vi "Command Loop - Set HW Values.vi"(8 "error in":errorcluster, 10 "Data":string, 11 "Queue Refs in":variant) -> (0 "error out":errorcluster, 2 "Response":string, 3 "Queue Refs out":variant)   [LabVIEW 2026, in "Runtime Configuration Support Example Engine.lvlib"]
uses:
  Runtime Configuration Support Example Engine.lvlib
  <vilib>/NI VeriStand/Custom Device API/Custom Device Item Ref.ctl
  <vilib>/NI VeriStand/Custom Device API/Custom Device API.lvlib
  Shared/Compiled.Settings.ctl
  Shared/Runtime Configuration Support Example Shared.lvlib
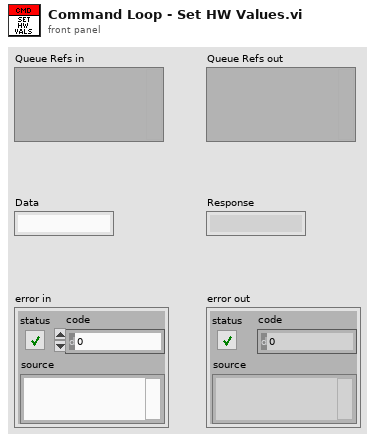
[diagram p1: front panel]
types:
  T1 = cluster{"Compiled Info":refnum<queue>, "Set HW Val Ref":refnum<queue>, "Get HW Val Ref":refnum<queue>}
  T2 = cluster{"SignalIDs":i32[], "Values":i32[], "Response Ref":refnum<queue>}
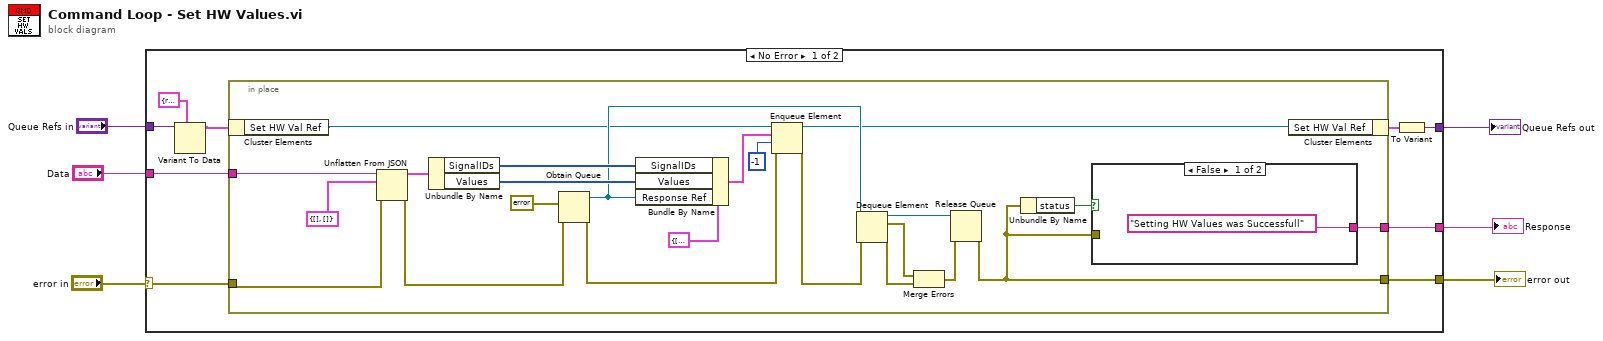
[diagram p0: block diagram]
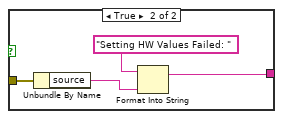
[diagram p2: hidden frame]
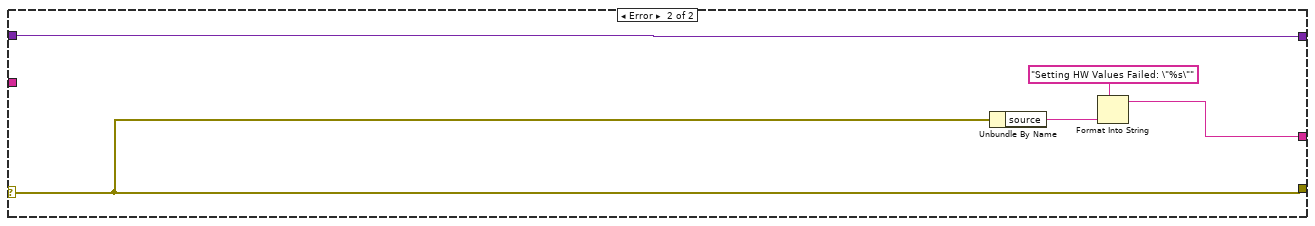
[diagram p3: hidden frame]
diagram:
  n1 = case shown="No Error" "error in" {
    selector: "error in" -> [w15 w48]
    tunnel: "Data" -> [w13 _]
    tunnel: "Queue Refs in" -> [w11 w44]
    tunnel: [w12 w45] -> w3
    tunnel: [w14 w48] -> w5
    tunnel: [w7 w44] -> w1
    frame No Error {
      n2 = Variant To Data(type=T1 {"Compiled Info"=refnum, "Set HW Val Ref"=refnum, "Get HW Val Ref"=refnum} ("Queue Refs in"), Variant=w11) -> (data=w10:T1)  [unwired: 1 in, 1 out]
      n3 = in-place {
        in-place-border: w15 -> [w34]
        in-place-border: [w32] -> w14
        in-place-border: w13 -> [w23]
        in-place-border: [w20] -> w12
        n4 = in-place-cluster #1(w10) -> ("Set HW Val Ref"=w19:refnum<queue>)
        n5 = Unflatten From JSON(JSON string=w23, type and defaults=cluster{"SignalIDs":i32[], "Values":i32[]} {"SignalIDs"=[], "Values"=[]} ("element"), error in (no error)=w34) -> (value=w26:cluster{"SignalIDs":i32[], "Values":i32[]}, error out=w30:errorcluster)  [unwired: 4 in]
        n6 = Unbundle By Name(w26) -> ("SignalIDs"=w27:i32[], "Values"=w28:i32[])
        n7 = Obtain Queue(element data type=errorcluster {"status"=FALSE, "code"=0, "source"=""} ("error constant"), error in (no error)=w30) -> (queue out=w22:refnum<queue>, error out=w35:errorcluster)  [unwired: 3 in, 1 out]
        n8 = Bundle By Name(cluster=T2 {"SignalIDs"=[], "Values"=[], "Response Ref"=refnum}, "SignalIDs"=w27, "Values"=w28, "Response Ref"=w22) -> (w25:T2)
        n9 = Enqueue Element(queue=w19, element=w25, timeout in ms (-1)=-1, error in (no error)=w35) -> (queue out=w18:refnum<queue>, error out=w31:errorcluster)  [unwired: 1 out]
        n10 = Dequeue Element(queue=w22, error in (no error)=w31) -> (queue out=w16:refnum<queue>, element=w38:errorcluster, error out=w37:errorcluster)  [unwired: 1 in, 1 out]
        n11 = Merge Errors(w38, w37) -> (w33:errorcluster)
        n12 = Release Queue(queue=w16, error in (no error)=w33) -> (error out=w32:errorcluster)  [unwired: 1 in, 2 out]
        n13 = Unbundle By Name(w32) -> ("status"=w21:bool)
        n14 = case shown="False" w21 {
          tunnel: ["Setting HW Values was Successfull" ("format string") w41] -> w20
          tunnel: w32 -> [_ w43]
          frame False {
          }
          frame True {
            n15 = Unbundle By Name(w43) -> ("source"=w42:string)
            n16 = Format Into String(initial string="Setting HW Values Failed: " ("format string"), w42) -> (resulting string=w41:string)  [unwired: 2 in, 1 out]
          }
        }
        n17 = in-place-cluster #1("Set HW Val Ref"=w18) -> (w8:T1)
      }
      n18 = To Variant(anything=w8) -> (Variant=w7:variant)
    }
    frame Error {
      n19 = Unbundle By Name(w48) -> ("source"=w46:string)
      n20 = Format Into String(format string="Setting HW Values Failed: \"%s\"", w46) -> (resulting string=w45:string)  [unwired: 2 in, 1 out]
    }
  }
  "error out" <- w5
  "Response" <- w3
  "Queue Refs out" <- w1
